vi "Change panel color.vi"(8 "error in":errorcluster, 10 "Pane Color":u32(colorbox), 11 "VI in":refnum<vi>) -> (0 "error out":errorcluster, 3 "VI out":refnum<vi>)   [LabVIEW 2019]
uses:
  <vilib>/Utility/traverseref.llb/TRef TravTarget.ctl
  <vilib>/Utility/traverseref.llb/VI Scripting - Traverse.lvlib
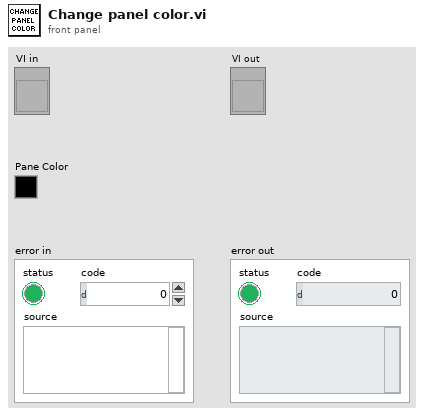
[diagram p1: front panel]
types:
  T1 = typedef "TRef TravTarget.ctl" = enum16{"FP", "BD", "Other"}
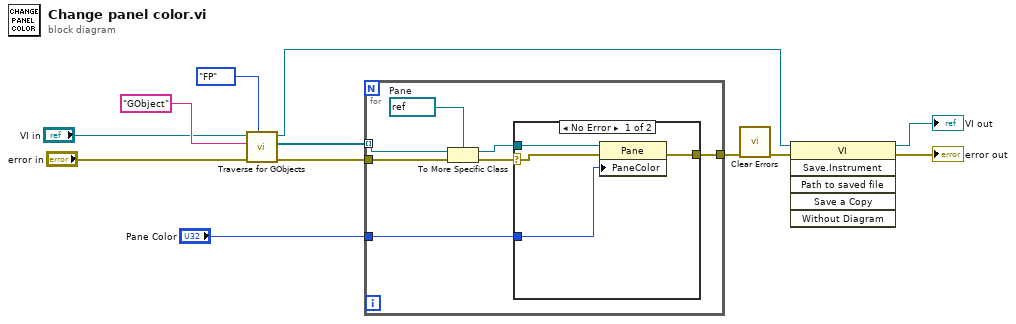
[diagram p0: block diagram]
diagram:
  n1 = call <vilib>:"Traverse for GObjects.vi"("Traverse Target"=TRef_TravTarget."FP", "error in (no error)"="error in", "Class Name"="GObject", "VI Refnum"="VI in") -> ("error out"=w10:errorcluster, "References"=w5:refnum<vi>[], "dup VI Refnum"=w6:refnum<vi>)  [unwired: 4 in, 1 out]
  n2 = for {
    tunnel: w5 -> [w16] mode=indexing
    tunnel: w10 -> [w18]
    tunnel: [w17] -> w11
    tunnel: "Pane Color" -> [w13]
    w15 = refnum<vi> refnum  # Pane
    n3 = To More Specific Class(target class=w15, reference=w16, error in=w18) -> (specific class reference=w14:refnum<vi>, error out=w19:errorcluster)
    n4 = case shown="No Error" w19 {
      selector: w19 -> [w23 w24]
      tunnel: w14 -> [w21 _]
      tunnel: [w22 w24] -> w17
      tunnel: w13 -> [w20 _]
      frame No Error {
        n5 = property class="Pane"(reference=w21, error in=w23, "PaneColor"=w20) -> (error out=w22:errorcluster)  [unwired: 1 out]
      }
      frame Error {
      }
    }
  }
  n6 = call <vilib>:"Clear Errors.vi"("error in (no error)"=w11) -> ("error out"=w12:errorcluster)  [unwired: 5 in, 1 out]
  n7 = invoke class="VI" method="Save.Instrument"(reference=w6, error in=w12) -> (reference out=→"VI out":refnum<vi>, error out=→"error out":errorcluster)  [unwired: 4 in, 4 out]
